vi "Read Current Position Array.vi"(8 "error in (no error)":errorcluster, 11 "Double Scanner in":refnum<class "Double Scanner.lvclass">) -> (0 "error out":errorcluster, 2 "Initial positions":dbl[](array[numeric]), 3 "Double Scanner out":refnum<class "Double Scanner.lvclass">)   [LabVIEW 2017, in "Double Scanner.lvclass"]
uses:
  Double Scanner.lvclass
  Scanner/Scanner.lvclass
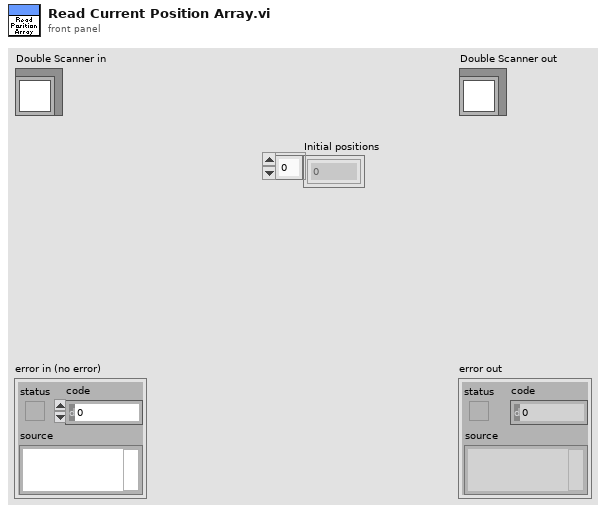
[diagram p1: front panel]
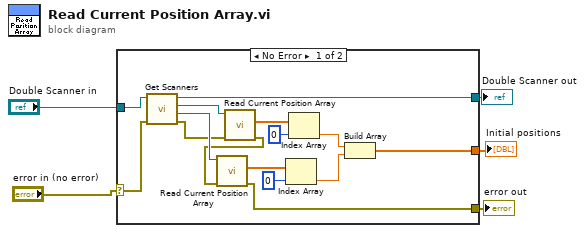
[diagram p0: block diagram]
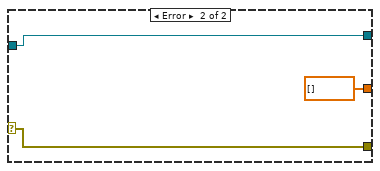
[diagram p2: hidden frame]
diagram:
  n1 = case shown="No Error" "error in (no error)" {
    selector: "error in (no error)" -> [w19 w22]
    tunnel: "Double Scanner in" -> [w20 w23]
    tunnel: [w7 w22] -> w3
    tunnel: [w18 w23] -> w2
    tunnel: [w13 dbl[] []] -> w1
    frame No Error {
      n2 = call-dynamic "Get Scanners.vi"("error in (no error)"=w19, "Double Scanner in"=w20) -> ("error out"=w10:errorcluster, "Scanner 2 out"=w11:refnum<class "Scanner.lvclass">, "Scanner 1 out"=w12:refnum<class "Scanner.lvclass">, "Double Scanner out"=w18:refnum<class "Double Scanner.lvclass">)  [unwired: 6 in]
      n3 = call-dynamic "Read Current Position Array.vi"("error in (no error)"=w10, "Scanner in"=w12) -> ("error out"=w6:errorcluster, "Position array"=w9:dbl[])  [unwired: 7 in, 1 out]
      n4 = call-dynamic "Read Current Position Array.vi"("error in (no error)"=w6, "Scanner in"=w11) -> ("error out"=w7:errorcluster, "Position array"=w8:dbl[])  [unwired: 7 in, 1 out]
      n5 = Index Array(array=w8, index=0) -> (element=w14:dbl)
      n6 = Index Array(array=w9, index=0) -> (element=w15:dbl)
      n7 = Build Array(w15, w14) -> (w13:dbl[])
    }
    frame Error {
    }
  }
  "error out" <- w3
  "Double Scanner out" <- w2
  "Initial positions" <- w1
